vi "residual_stress_calc.vi"(1 "DiamCorrigido":dbl, 2 "Pasta das imagens":path=path "C:/Users/l01481/Documents/Serviços já concluidos/Tensão residual/Molas Volvo/Imagens Volvo", 3 "Pasta do ensaio":path=path "L:/Documentos/Serviços já concluidos/Tensão residual/Molas Volvo/Dados/Terceiro grupo/Amostra_1_0") -> (0 "ResultsDist":dbl[](array[numeric]))   [LabVIEW 2016]
panel:
  in  "Tab Control":T1(tab)
  in  "R (E2/E1)":dbl=0.1
  in  "Sesc":dbl=600.0 caption="Tensão de escoamento [MPa]"
  out "Uniformidade":cluster{"Array":dbl[], "Array":dbl[]}[](graph)
  out "C plast":cluster{"Resultados":dbl[], dbl[]}[](graph) caption="Correção plasticidade"
  out "Resultados médios":string[][](table)
  out "Resultados":string[][](table)
  out "Dados":T2
  # "Programa de processamento para Tensão Residual"
  # "Diâmetro da roseta"
  # "Dados para correção da plasticidade\nModelo Bilinear"
  # "Equações"
  # "P, Q e T são combinações das deformações medidas ponderadas pelos coeficientes da norma"
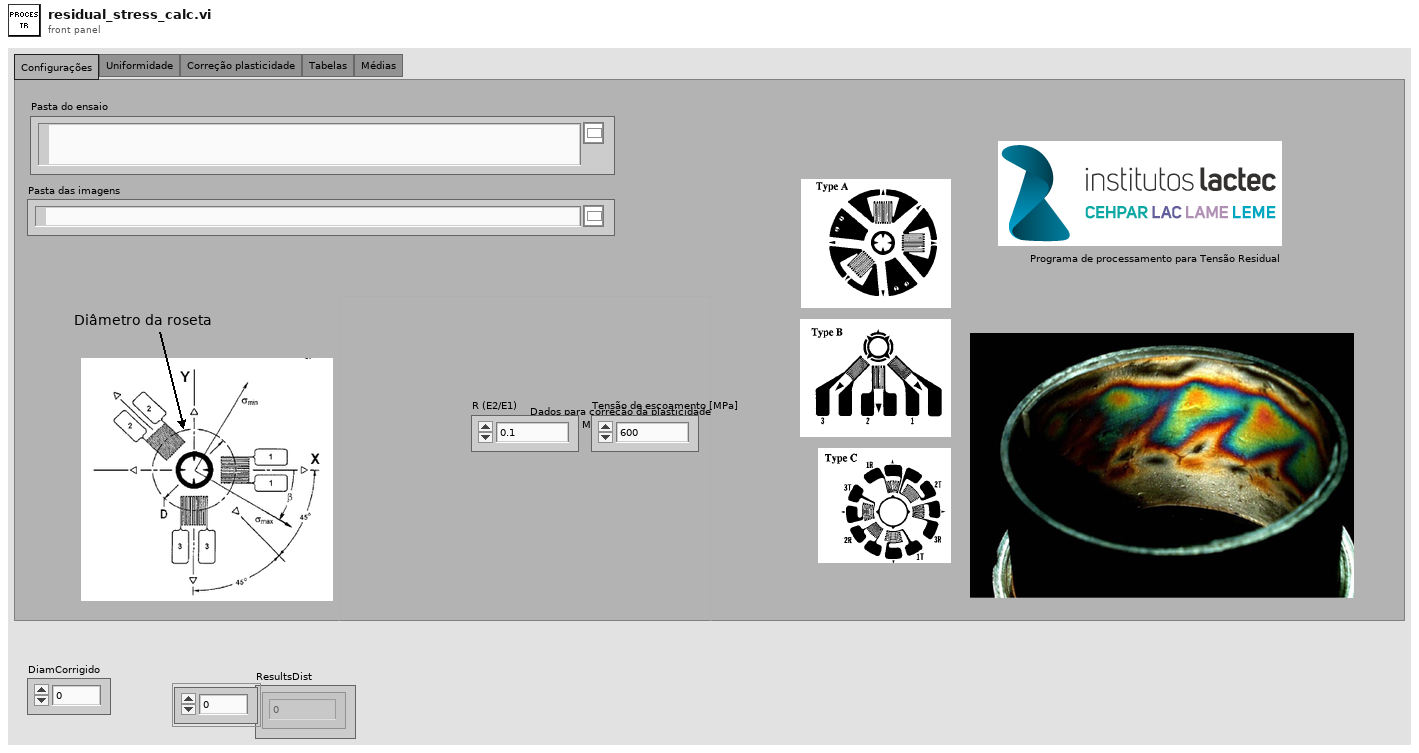
[diagram p1: front panel]
types:
  T1 = enum32{"Configurações", "Uniformidade", "Correção plasticidade", "Tabelas", "Médias"}
  T2 = typedef "Deformações.ctl" = cluster{"def. 1 ":dbl[], "def. 2":dbl[], "def. 3":dbl[], "z":dbl[]}
  T3 = typedef "Infos para processamento.ctl" = cluster{"Diâmetro do furo [mm]":dbl, "Diâmetro da linha média [mm]":dbl, "IncF":dbl, "Módulo de elasticidade [GPa]":dbl, "Módulo de Poisson":dbl, "Tipo de roseta utilizada":enum16{"Tipo A", "Tipo B", "Tipo C"}, "Método de análise":enum16{"Não uniforme 2013", "Simplificado 2013", "Simplificado 2008"}, "Pfinal":dbl, "Parar auto.":bool}
  T4 = typedef "p,q, t, a e b.ctl" = cluster{"p":dbl[], "q":dbl[], "t":dbl[], "z":dbl[], "a":dbl[], "b":dbl[]}
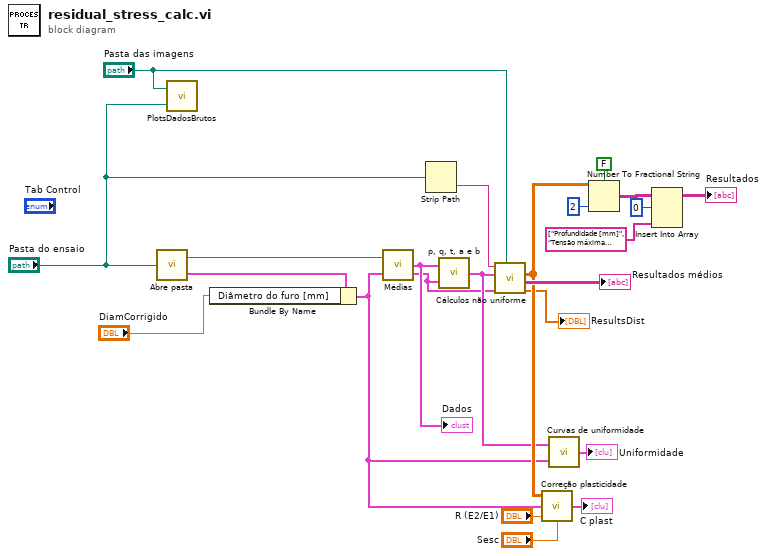
[diagram p0: block diagram]
diagram:
  n1 = call "Abre pasta.vi"("Pasta do ensaio"="Pasta do ensaio") -> ("Dados"=w22:string, "Infos para processamento out"=w7:T3)
  n2 = call "PlotsDadosBrutos.vi"("Pasta do ensaio"="Pasta do ensaio", "Pasta das imagens"="Pasta das imagens") -> ()  [unwired: 1 in]
  n3 = Bundle By Name(cluster=w7, "Diâmetro do furo [mm]"="DiamCorrigido") -> (w5:T3)
  n4 = call "Médias.vi"("Infos para processamento"=w5, "Dados"=w22) -> ("Dados"=w13:T2)
  "Dados" <- w13
  n5 = Strip Path(path="Pasta do ensaio") -> (name=w1:string)  [unwired: 1 out]
  n6 = call "p, q, t, a e b.vi"("Infos para processamento"=w5, "Dados in"=w13) -> ("Dados out"=w9:T4)
  n7 = call "Cálculos não uniforme.vi"("PathImagem"="Pasta das imagens", "Infos para processamento in"=w5, "Dados in"=w9, "Tag"=w1) -> ("ResultsDist"=→"ResultsDist":dbl[], "Resultados médios"=→"Resultados médios":string[][], "Resultados"=w20:dbl[][])  [unwired: 2 in]
  n8 = call "Correção plasticidade.vi"("Sesc"="Sesc", "R"="R (E2/E1)", "Infos para processamento"=w5, "Resultados"=w20) -> ("Comparação"=→"C plast":cluster{"Resultados":dbl[], dbl[]}[])
  n9 = call "Curvas de uniformidade.vi"("Infos para processamento"=w5, "Dados out"=w9) -> ("Gráficos"=→"Uniformidade":cluster{"Array":dbl[], "Array":dbl[]}[])
  n10 = Number To Fractional String(use system decimal point (T)=FALSE, number=w20, precision (6)=i16 2) -> (F-format string=w17:string[][])  [unwired: 1 in]
  n11 = Insert Into Array(array=w17, index (row)=0, new element=string[] ["Profundidade [mm]", "Tensão máxima [MPa]", "Tensão mínima [MPa]", "Tensão em x [MPa]", "Tensão em y [MPa]", "Tensão cisalhante [MPa]", "Ângulo da tensão máxima [°]", "Tensão de Von Misses [MPa]"] ("new element/subarray")) -> (→"Resultados":string[][])  [unwired: 1 in]
